vi "defuzzy.vi"(0 "Controller":T2={"Parameters"={"antecedance"=[{"ling.var."="in1", "x-min"=-1.0, "x-max"=1.0, "setarray"=[{"linguistic term"="NE1", "color"=16711680, "points"=[-1.0, -1.0, -1.0, -2.2351741790771484e-05]}, {"linguistic term"="ZE1", "color"=255, "points"=[-1.0, 0.0, 0.0, 1.0]}, {"linguistic term"="PO1", "color"=26214, "points"=[0.0, 1.0, 1.0, 1.0]}]}, {"ling.var."="in2", "x-min"=-1.0, "x-max"=1.0, "setarray"=[{"linguistic term"="NE2", "color"=16711680, "points"=[-1.0, -1.0, -1.0, 0.0]}, {"linguistic term"="ZE2", "color"=255, "points"=[-1.0, 0.0, 0.0, 1.0]}, {"linguistic term"="PO2", "color"=26214, "points"=[0.0, 1.0, 1.0, 1.0]}]}], "consequence"=[{"ling.var."="out", "x-min"=-1.0, "x-max"=1.0, "setarray"=[{"linguistic term"="NEo", "color"=16711680, "points"=[-1.0, -1.0, -1.0, 0.0]}, {"linguistic term"="ZEo", "color"=255, "points"=[-1.0, 0.0, 0.0, 1.0]}, {"linguistic term"="POo", "color"=26214, "points"=[0.0, 1.0, 1.0, 1.0]}]}], "conclusions"=[3, 3, 3, 3, 3, 3, 3], "degree-of-support"=[1.0, 1.0, 1.0, 1.0, 1.0, 1.0, 1.0], "defu"=[{"inference"=0, "defumethod"=0, "modification"=TRUE, "precision"=0, "no consequence"=0, "defaultvalue"=0.0}]}, "Description"={"Info"={"Path"=path "/HD 1000/Desktop Folder/fuzzylab today/loadsave.vi", "Controller Name"="", "Date"="", "Time"=""}, "Author"="", "Text"=""}} {"Parameters"."defu"."defaultvalue" format="%.2f"; "Parameters"."degree-of-support" step=0.009999999776482582 format="%.2f"; "Parameters"."consequence"."x-min" step=0.009999999776482582 format="%.2f"; "Parameters"."consequence"."x-max" step=0.009999999776482582 format="%.2f"; "Parameters"."consequence"."setarray"."points" step=0.009999999776482582 format="%.2f"; "Parameters"."antecedance"."x-min" step=0.009999999776482582 format="%.2f"; "Parameters"."antecedance"."x-max" step=0.009999999776482582 format="%.2f"; "Parameters"."antecedance"."setarray"."points" step=0.009999999776482582 format="%.2f"}, 1 "inference results":T1={"fullfilment*DoS"=[0.0, 0.25, 0.75], "active consequence"=[0, 1, 2]} {"fullfilment*DoS" step=0.01 format="%.2f"}) -> (2 "analog output":dbl=-1.0 format="%.2f", 3 "output assessment":string, 4 "error out":errorcluster)   [LabVIEW 2020, in "NI_fuzzy logic.lvlib"]
uses:
  <vilib>/addons/control/fuzzy/NI_fuzzy logic.lvlib
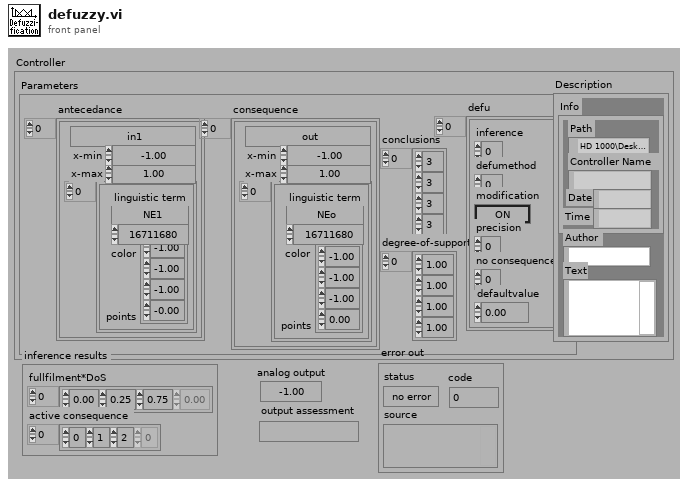
[diagram p1: front panel]
types:
  T1 = cluster{"fullfilment*DoS":dbl[], "active consequence":i32[]}
  T2 = cluster{"Parameters":cluster{"antecedance":cluster{"ling.var.":string, "x-min":dbl, "x-max":dbl, "setarray":cluster{"linguistic term":string, "color":u32, "points":dbl[]}[]}[], "consequence":cluster{"ling.var.":string, "x-min":dbl, "x-max":dbl, "setarray":cluster{"linguistic term":string, "color":u32, "points":dbl[]}[]}[], "conclusions":u16[], "degree-of-support":dbl[], "defu":cluster{"inference":u16, "defumethod":u16, "modification":bool, "precision":u16, "no consequence":u16, "defaultvalue":dbl}[]}, "Description":cluster{"Info":cluster{"Path":path, "Controller Name":string, "Date":string, "Time":string}, "Author":string, "Text":string}}
  T3 = cluster{"ling.var.":string, "x-min":dbl, "x-max":dbl, "setarray":cluster{"linguistic term":string, "color":u32, "points":dbl[]}[]}[]
  T4 = cluster{"inference":u16, "defumethod":u16, "modification":bool, "precision":u16, "no consequence":u16, "defaultvalue":dbl}[]
  T5 = cluster{"inference":u16, "defumethod":u16, "modification":bool, "precision":u16, "no consequence":u16, "defaultvalue":dbl}
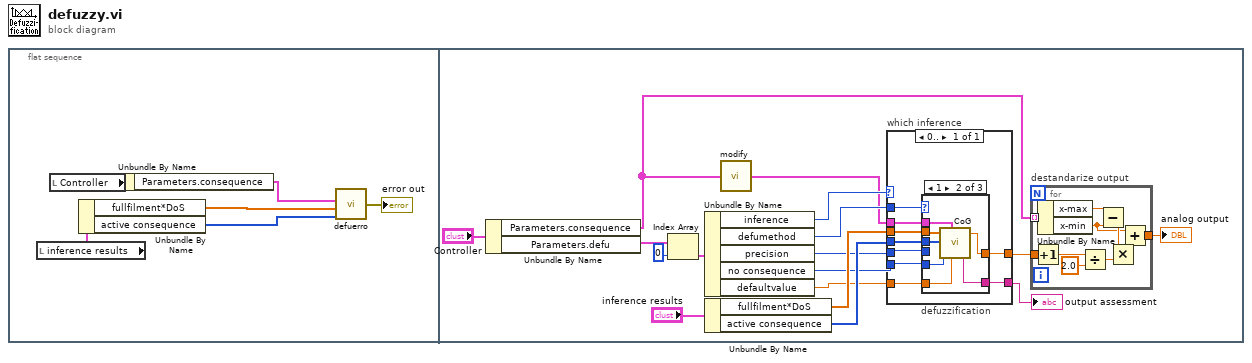
[diagram p0: block diagram]
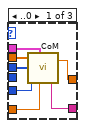
[diagram p2: hidden frame]
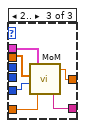
[diagram p3: hidden frame]
diagram:
  n1 = flat-sequence {
    frame #0 {
      n2 = local read "inference results"() -> (w3:T1)
      n3 = local read "Controller"() -> (w5:T2)
      n4 = Unbundle By Name(w3) -> ("fullfilment*DoS"=w2:dbl[], "active consequence"=w1:i32[])
      n5 = Unbundle By Name(w5) -> ("Parameters.consequence"=w4:T3)
      n6 = call <vilib>:"defuerro.vi"("active consequence"=w1, "fullfilment consequence"=w2, "consequence"=w4) -> ("error out"=→"error out":errorcluster)  [unwired: 1 out]
    }
    frame #1 {
      n7 = Unbundle By Name("Controller") -> ("Parameters.consequence"=w7:T3, "Parameters.defu"=w9:T4)
      n8 = Index Array(array=w9, index=0) -> (element=w11:T5)
      n9 = Unbundle By Name(w11) -> ("inference"=w14:u16, "defumethod"=w23:u16, "precision"=w17:u16, "no consequence"=w15:u16, "defaultvalue"=w16:dbl)
      n10 = Unbundle By Name("inference results") -> ("fullfilment*DoS"=w22:dbl[], "active consequence"=w21:i32[])
      n11 = call <vilib>:"modify.vi"("consequence"=w7) -> ("consequence modified"=w8:T3)
      n12 = case "which inference" shown="0.." w14 {
        tunnel: [w32] -> w18
        tunnel: w8 -> [w31]
        tunnel: w22 -> [w30]
        tunnel: w21 -> [w29]
        tunnel: w23 -> [w28]
        tunnel: w17 -> [w27]
        tunnel: w15 -> [w26]
        tunnel: w16 -> [w25]
        tunnel: [w24] -> w20
        frame 0.. {
          n13 = case "defuzzification" shown="1" w28 {
            tunnel: w31 -> [w39 w45 w52]
            tunnel: [w34 w41 w47] -> w32
            tunnel: w30 -> [w38 w46 w51]
            tunnel: w29 -> [w37 w44 _]
            tunnel: w27 -> [_ _ _]
            tunnel: w26 -> [w36 w43 w50]
            tunnel: w25 -> [w35 w42 w49]
            tunnel: [w33 w40 w48] -> w24
            frame ..0 {
              n14 = call <vilib>:"CoM.vi"("fullfilment consequence"=w38, "consequence"=w39, "active consequence"=w37, "output when no consequence (0)"=w36, "output default (0,00)"=w35) -> ("controller output"=w34:dbl, "output assessment"=w33:string)
            }
            frame 1 {
              n15 = call <vilib>:"CoG.vi"("fullfilment consequence"=w46, "consequence"=w45, "active consequence"=w44, "output when no consequence (0)"=w43, "output default (0,00)"=w42) -> ("controller output"=w41:dbl, "output assessment"=w40:string)
            }
            frame 2.. {
              n16 = call <vilib>:"MoM.vi"("outputterm default (0)"=w49, "output when no consequence (0)"=w50, "fullfilment consequence"=w51, "consequence"=w52) -> ("output assessment"=w48:string, "controller output"=w47:dbl)
            }
          }
        }
      }
      "output assessment" <- w20
      n17 = for "destandarize output" {
        tunnel: w7 -> [w62] mode=indexing
        tunnel: w18 -> [w60]
        tunnel: [w53] -> w19
        n18 = Increment(x=w60) -> (x+1=w58:dbl)
        n19 = Unbundle By Name(w62) -> ("x-max"=w61:dbl, "x-min"=w54:dbl)
        n20 = Divide(x=w58, y=2.0) -> (x/y=w57:dbl)
        n21 = Subtract(x=w61, y=w54) -> (x-y=w56:dbl)
        n22 = Multiply(x=w56, y=w57) -> (x*y=w55:dbl)
        n23 = Add(x=w54, y=w55) -> (x+y=w53:dbl)
      }
      "analog output" <- w19
    }
  }
